vi "Initialize 5R Type 1 Serial Arm.vi"(6 "L4":dbl=0.1136 format="%#_13g", 7 "L3":dbl=0.135, 8 "error in (no error)":errorcluster, 9 "L2":dbl=0.155, 10 "L1z":dbl=0.11, 11 "L1x":dbl=0.033) -> (0 "error out":errorcluster, 3 "5R type 1 serial arm out":refnum<class "NI_Robotics_5R Type 1 Serial Arm Class.lvclass">)   [LabVIEW 2017, in "NI_Robotics_5R Type 1 Serial Arm Class.lvclass"]
doc: "Sets the properties of a serial robot arm and generates a representation of the arm. If you have access to a 6R, 5R, or SCARA arm, generate that type of arm. If you do not have access to an arm of those types, generate a generic arm. You must manually select the polymorphic instance to use."
uses:
  <vilib>/robotics/Kinematics/Analytical/5R/Type 1/NI_Robotics_5R Type 1 Serial Arm Class.lvclass
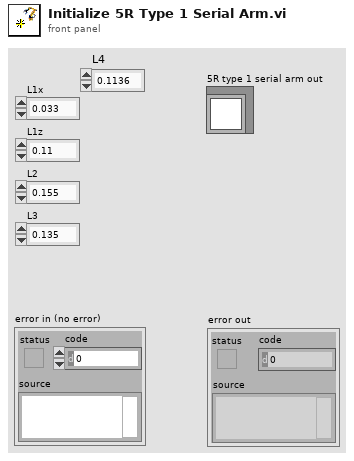
[diagram p1: front panel]
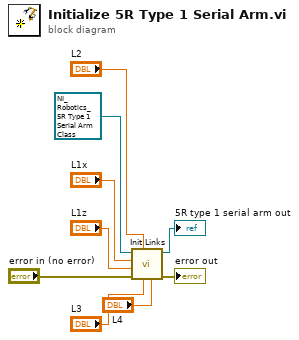
[diagram p0: block diagram]
diagram:
  n1 = call-dynamic "Init Links.vi"("L4"="L4", "L3"="L3", "L2"="L2", "error in (no error)"="error in (no error)", "L1z"="L1z", "L1x"="L1x", "NI_Robotics_5R Type 1 Serial Arm Class in"=refnum<class "NI_Robotics_5R Type 1 Serial Arm Class.lvclass"> refnum ("NI_Robotics_5R Type 1 Serial Arm Class.lvclass")) -> ("error out"=→"error out":errorcluster, "NI_Robotics_5R Type 1 Serial Arm Class out"=→"5R type 1 serial arm out":refnum<class "NI_Robotics_5R Type 1 Serial Arm Class.lvclass">)  [unwired: 3 in]
